vi "ECGfirst.vi"() -> ()   [LabVIEW 2015]
uses:
  <vilib>/Instr/_visa.llb/VISA Configure Serial Port (Instr).vi
panel:
  out "Serial Settings:Number of Bytes at Serial Port":u32
  in  "Menus":enum32{"Configuración", "Variables", "Graficas"}(tab)
  in  "Text & Pict Ring 2":u16(ring) items=["Tiempo Real"=1, "Desconectado"=2, "Datos almaceados"=3, "Alarma Medir"=0]
  in  "LECTURA":bool
  in  "ESCRITURA":bool
  in  "Stop Button 2":bool
  in  "VISA resource name":refnum<visa-resource-name>
  out "read buffer":string
  out "Numeric":dbl
  out "Al PIC":string
  out "Array":dbl[](array[numeric])
  out "Waveform Chart":dbl(graph)
  # "ELECTROCARDIOGRAFO \nPORTATIL"
  # "(Seg)"
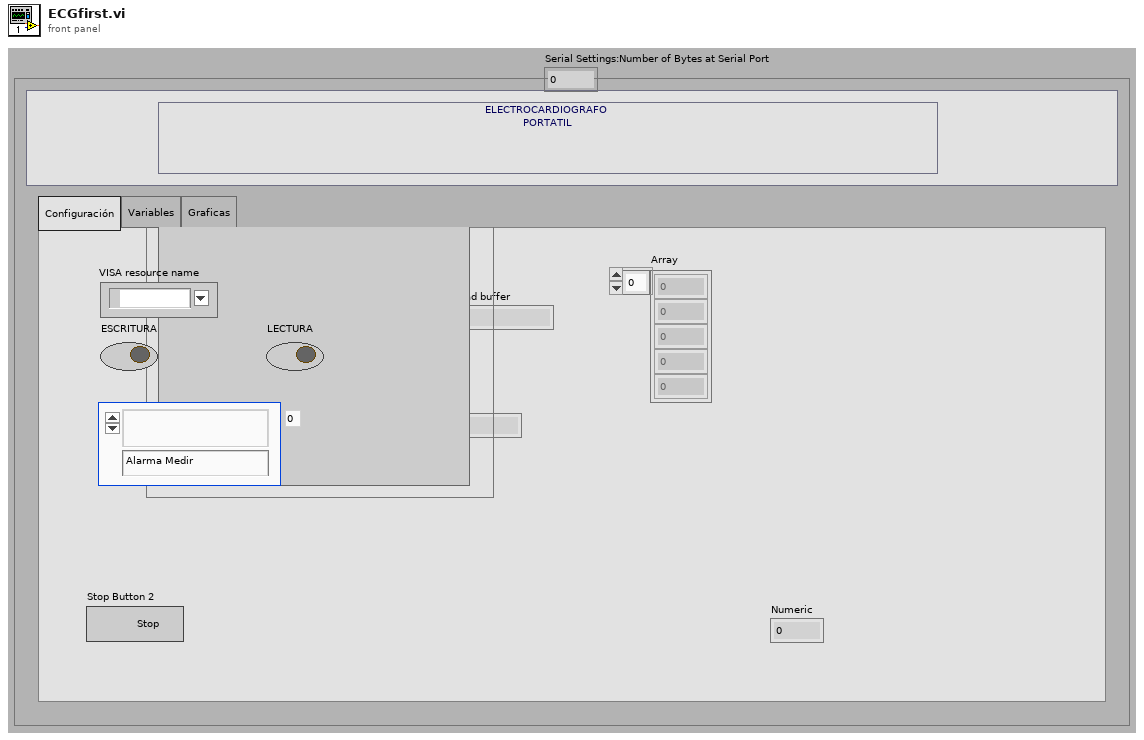
[diagram p1: front panel]
types:
  T1 = cluster{"unsigned byte array[0]":u8, "unsigned byte array[1]":u8, "unsigned byte array[2]":u8, "unsigned byte array[3]":u8, "unsigned byte array[4]":u8, "unsigned byte array[5]":u8, "unsigned byte array[6]":u8, "unsigned byte array[7]":u8, "unsigned byte array[8]":u8}
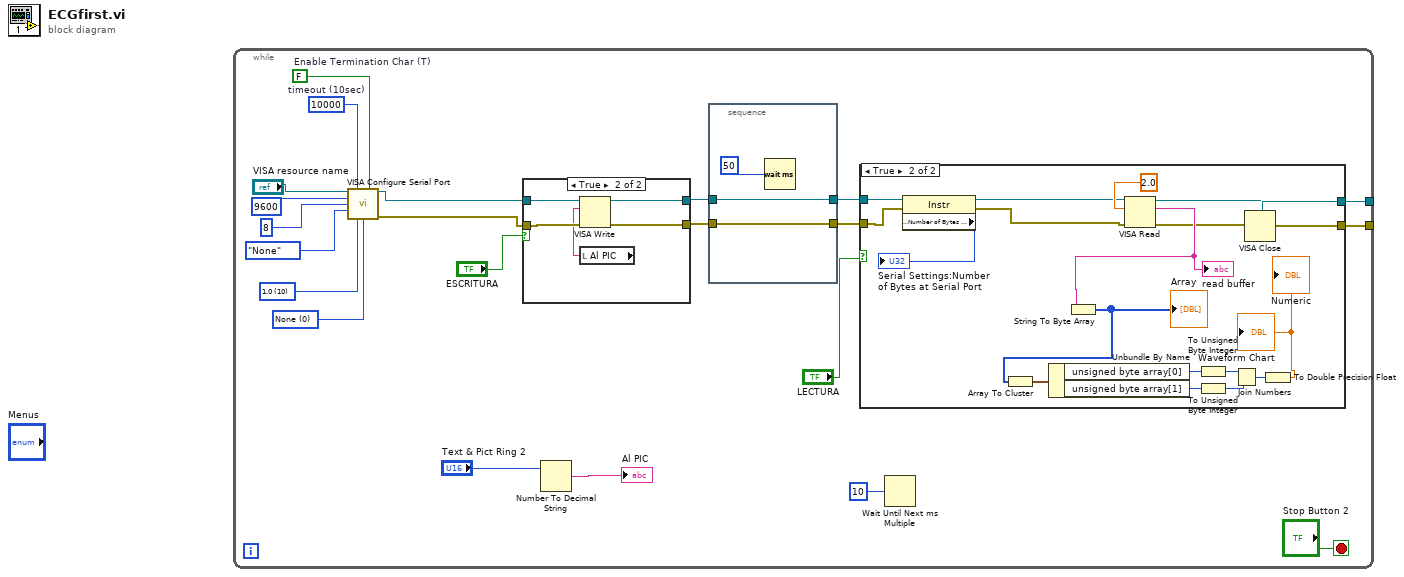
[diagram p0: block diagram]
diagram:
  n1 = while {
    tunnel: [w24] -> w2
    tunnel: [w23] -> w1
    stop <- "Stop Button 2" stop-if-true
    w14 = u16 0 items=["None", "XON/XOFF", "RTS/CTS", "XON/XOFF & RTS/CTS", "DTR/DSR", "XON/XOFF & DTR/DSR"] ("flow control (0:none)")
    w13 = FALSE  # Enable Termination Char (T)
    w12 = u32 10000  # timeout (10sec)
    w9 = u16 10 items=["1.0"=10, "1.5"=15, "2.0"=20] ("stop bits (10: 1 bit)")
    n2 = call-poly "VISA Configure Serial Port"("VISA resource name"="VISA resource name", "timeout (10sec)"=w12, "Enable Termination\nChar (T)"=w13, "baud rate (9600)"=9600 ("Numeric 2"), "data bits (8)"=u16 8, "parity (0:none)"=enum16{"None", "Odd", "Even", "Mark", "Space"}."None", "stop bits (10: 1 bit)"=w9, "flow control (0:none)"=w14) -> ("VISA resource name out"=w6:refnum<visa-resource-name>, "error out"=w5:errorcluster)  [unwired: 6 in]
    n3 = case shown="True" "ESCRITURA" {
      tunnel: w6 -> [w48 w53]
      tunnel: [w48 w49] -> w19
      tunnel: [w47 w52] -> w18
      tunnel: w5 -> [w47 w51]
      frame False {
      }
      frame True {
        n4 = local read "Al PIC"() -> (w50:string)
        n5 = VISA Write(VISA resource name=w53, write buffer=w50, error in (no error)=w51) -> (VISA resource name out=w49:refnum<visa-resource-name>, error out=w52:errorcluster)  [unwired: 1 out]
      }
    }
    n6 = Number To Decimal String(number="Text & Pict Ring 2") -> (decimal integer string=→"Al PIC":string)  [unwired: 1 in]
    n7 = stacked-sequence {
      tunnel: w18 -> [w27]
      tunnel: [w27] -> w16
      tunnel: w19 -> [w26]
      tunnel: [w26] -> w17
      frame #0 {
        n8 = Wait (ms)(milliseconds to wait=u32 50 ("delay before\nread (ms)")) -> ()  [unwired: 1 out]
      }
    }
    n9 = case shown="True" "LECTURA" {
      tunnel: w17 -> [w29 w34]
      tunnel: [w29 w36] -> w24
      tunnel: [w28 w35] -> w23
      tunnel: w16 -> [w28 w32]
      frame False {
      }
      frame True {
        n10 = property class="Instr"(reference=w34, error in=w32) -> (reference out=w33:refnum<visa-resource-name>, error out=w31:errorcluster, "Serial Settings:Number of Bytes at Serial Port"=→"Serial Settings:Number of Bytes at Serial Port":u32)
        n11 = VISA Read(VISA resource name=w33, byte count=2.0 ("BYTES A LEER"), error in (no error)=w31) -> (VISA resource name out=w36:refnum<visa-resource-name>, read buffer=w46:string, error out=w35:errorcluster)  [unwired: 1 out]
        "read buffer" <- w46
        n12 = String To Byte Array(string=w46) -> (unsigned byte array=w37:u8[])
        "Array" <- w37
        n13 = Array To Cluster(array=w37) -> (cluster=w45:T1)
        n14 = Unbundle By Name(w45) -> ("unsigned byte array[0]"=w41:u8, "unsigned byte array[1]"=w40:u8)
        n15 = To Unsigned Byte Integer(number=w41) -> (unsigned 8bit integer=w44:u8)
        n16 = To Unsigned Byte Integer(number=w40) -> (unsigned 8bit integer=w43:u8)
        n17 = Join Numbers(hi=w44, lo=w43) -> ((hi.lo)=w42:u16)
        n18 = To Double Precision Float(number=w42) -> (double precision float=→"Numeric" →"Waveform Chart":dbl)
      }
    }
    n19 = Wait Until Next ms Multiple(millisecond multiple=u32 10 ("Vielfache von ms")) -> ()  [unwired: 1 out]
  }
  n20 = VISA Close(VISA resource name=w2, error in (no error)=w1) -> ()  [unwired: 1 out]
